vi "Gmsg_RR_Handler.vi"() -> ()   [LabVIEW 2013]
uses:
  source/actor/Reply/FTW-Reply.lvclass
  source/actor/Message/Request/FTW-Message-IncomingRequest.lvclass
panel:
  out "Actual Address":string
  in  "Connection":string(combo)="tcp://localhost:51213"
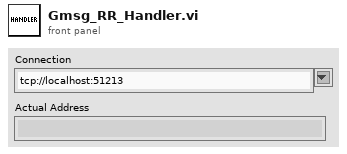
[diagram p1: front panel]
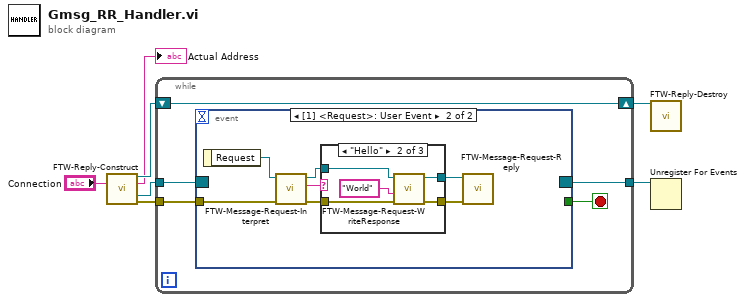
[diagram p0: block diagram]
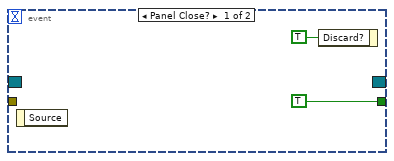
[diagram p2: hidden frame]
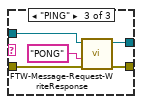
[diagram p4: hidden frame]
diagram:
  n1 = call "FTW-Reply-Construct.vi"("Address"="Connection") -> ("FTW-Router Out"=w6:refnum<class "FTW-Reply.lvclass">, "Actual Address"=→"Actual Address":string, "Event Registration Refnum"=w3:refnum<event-registration>, "error out"=w5:errorcluster)  [unwired: 11 in]
  n2 = while {
    tunnel: w3 -> [w11]
    tunnel: [w10] -> w7
    shift-right: [w8] -> w4
    shift-left: w6 -> [w8]
    tunnel: w5 -> [w9]
    stop <- w12 stop-if-true
    n3 = event shown="[1] <Request>: User Event" {
      selector: w11 -> [_ _]
      dyn-events: [_ _] -> w10
      timeout: _ -> [_ _]
      tunnel: [TRUE _] -> w12
      tunnel: w9 -> [_ w21]
      event Panel Close? {
        n4 = event-data() -> ()  [unwired: 1 in, 1 out]
        n5 = event-data("Discard?"=TRUE) -> ()  [unwired: 1 in, 1 out]
      }
      event User Event {
        n6 = event-data() -> ("Request"=w20:refnum<class "FTW-Message-IncomingRequest.lvclass">)  [unwired: 1 in]
        n7 = call "FTW-Message-Request-Interpret.vi"("error in"=w21, "FTW Incoming Request"=w20) -> ("error out"=w15:errorcluster, "Request Header"=w19:string, "FTW Incoming Request out"=w18:refnum<class "FTW-Message-IncomingRequest.lvclass">)  [unwired: 7 in]
        n8 = case shown="\"Hello\"" w19 {
          tunnel: w18 -> [w23 w26 w31]
          tunnel: [w23 w25 w30] -> w17
          tunnel: [w22 w27 w32] -> w16
          tunnel: w15 -> [w22 w28 w33]
          frame "False", Default {
          }
          frame "Hello" {
            n9 = call "FTW-Message-Request-WriteResponse.vi"("error in"=w28, "Response Body"="World", "FTW Incoming Request"=w26) -> ("error out"=w27:errorcluster, "FTW Incoming Request out"=w25:refnum<class "FTW-Message-IncomingRequest.lvclass">)  [unwired: 7 in]
          }
          frame "PING" {
            n10 = call "FTW-Message-Request-WriteResponse.vi"("error in"=w33, "Response Body"="PONG", "FTW Incoming Request"=w31) -> ("error out"=w32:errorcluster, "FTW Incoming Request out"=w30:refnum<class "FTW-Message-IncomingRequest.lvclass">)  [unwired: 7 in]
          }
        }
        n11 = call "FTW-Message-Request-Reply.vi"("error in"=w16, "FTW Incoming Request"=w17) -> ()  [unwired: 8 in, 2 out]
      }
    }
  }
  n12 = call "FTW-Reply-Destroy.vi"("FTW-Router In"=w4) -> ()  [unwired: 14 in, 1 out]
  n13 = Unregister For Events(event registration refnum=w7) -> ()  [unwired: 1 in, 1 out]
